vi "TEST - Get Array Element TDEnum.vi"(8 "error in (no error)":errorcluster) -> (0 "error out":errorcluster, 2 "pass":bool)   [LabVIEW 2013]
uses:
  source/library/Type Descriptor Enumeration.ctl
panel:
  out "Failures":T2(array[cluster]) {"result"."Element Type" format="%.0x"; "exected result"."Element Type" format="%.0x"}
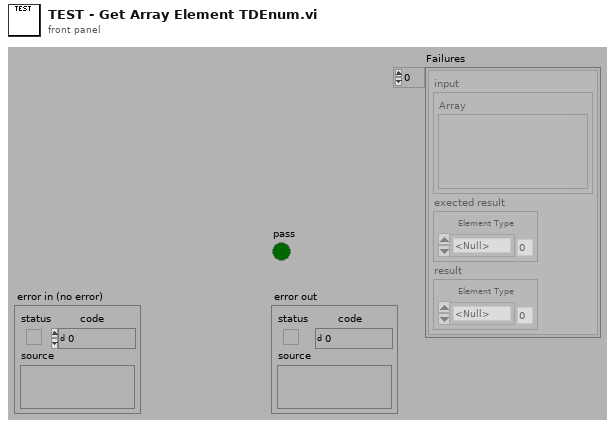
[diagram p1: front panel]
types:
  T1 = typedef "Type Descriptor Enumeration.ctl" = enum8{"<Null>", "I8", "I16", "I32", "I64", "U8", "U16", "U32", "U64", "SGL", "DBL", "EXT", "CSG", "CDB", "CXT", "0x0F", "0x10", "0x11", "0x12", "0x13", "0x14", "Enum U8", "Enum U16", "Enum U32", "Enum U64", "SGL PQ", "DBL PQ", "EXT PQ", "CSG PQ", "CDB PQ", "CXT PQ", "0x1F", "0x20", "Boolean", "0x22", "0x23", "0x24", "0x25", "0x26", "0x27", "0x28", "0x29", "0x2A", "0x2B", "0x2C", "0x2D", "0x2E", "0x2F", "String", "0x31", "Path", "Pict", "0x34", "0x35", "0x36", "DAQ", "0x38", "0x39", "0x3A", "0x3B", "0x3C", "0x3D", "0x3E", "0x3F", "Array", "0x41", "0x42", "0x43", "0x44", "0x45", "0x46", "0x47", "0x48", "0x49", "0x4A", "0x4B", "0x4C", "0x4D", "0x4E", "0x4F", "Cluster", "0x51", "0x52", "Variant", "Waveform", "0x55", "0x56", "0x57", "0x58", "0x59", "0x5A", "0x5B", "0x5C", "0x5D", "0x5E", "0x5F", "0x60", "0x61", "0x62", "0x63", "0x64", "0x65", "0x66", "0x67", "0x68", "0x69", "0x6A", "0x6B", "0x6C", "0x6D", "0x6E", "0x6F", "Refnum"}
  T2 = cluster{"input":cluster{"Array":variant}, "exected result":cluster{"Element Type":T1}, "result":cluster{"Element Type":T1}}[]
  T3 = typedef "Type Descriptor Header.ctl" = cluster{"length":u16, "private":u8, "type":T1, "# elements":u16}
  T4 = cluster{"input":cluster{"Array":variant}, "exected result":cluster{"Element Type":T1}, "result":cluster{"Element Type":T1}}
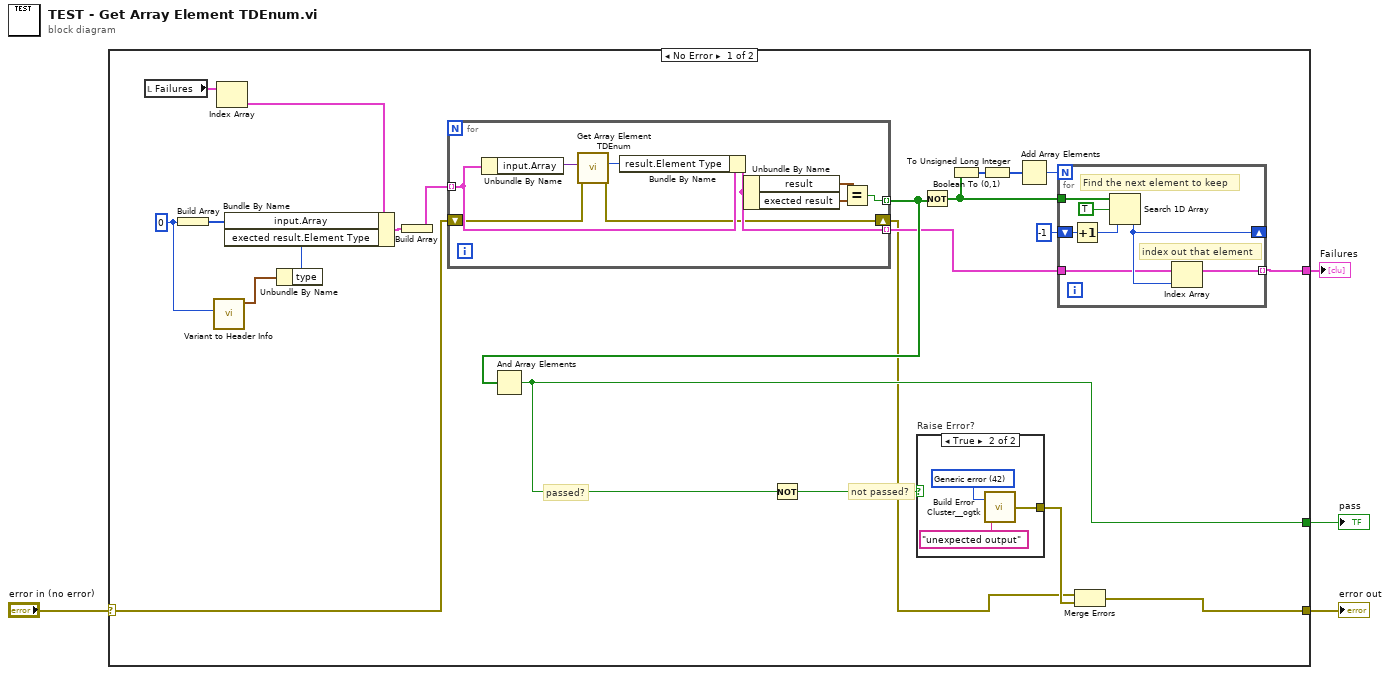
[diagram p0: block diagram]
diagram:
  n1 = case shown="No Error" "error in (no error)" {
    selector: "error in (no error)" -> [w12 w46]
    tunnel: [w23 _] -> w4
    tunnel: [w26 w46] -> w2
    tunnel: [w15 _] -> w1
    frame No Error {
      w6 = 0
      # "not passed?"
      # "passed?"
      n2 = local read "Failures"() -> (w10:T2)
      n3 = Build Array(w6) -> (w8:i32[])
      n4 = call "Variant to Header Info.vi"("Variant"=w6) -> ("Type Descriptor Header"=w7:T3)  [unwired: 3 in, 2 out]
      n5 = Index Array(array=w10) -> (element=w9:T4)  [unwired: 1 in]
      n6 = Unbundle By Name(w7) -> ("type"=w5:T1)
      n7 = Bundle By Name(cluster=w9, "input.Array"=w8, "exected result.Element Type"=w5) -> (w14:T4)
      n8 = Build Array(w14) -> (w13:T2)
      n9 = for {
        tunnel: w13 -> [w41] mode=indexing
        tunnel: [w42] -> w17 mode=indexing
        tunnel: [w40] -> w16 mode=indexing
        shift-right: [w34] -> w11
        shift-left: w12 -> [w35]
        n10 = Unbundle By Name(w41) -> ("input.Array"=w37:variant)
        n11 = call "Get Array Element TDEnum.vi"("error in (no error)"=w35, "Array"=w37) -> ("error out"=w34:errorcluster, "Element Type"=w36:T1)  [unwired: 8 in]
        n12 = Bundle By Name(cluster=w41, "result.Element Type"=w36) -> (w40:T4)
        n13 = Unbundle By Name(w40) -> ("result"=w39:cluster{"Element Type":T1}, "exected result"=w38:cluster{"Element Type":T1})
        n14 = Equal?(x=w39, y=w38) -> (x = y?=w42:bool)
      }
      n15 = And Array Elements(Boolean array=w17) -> (logical AND=w23:bool)
      n16 = Not(x=w23) -> (.not. x?=w24:bool)
      n17 = case "Raise Error?" shown="True" w24 {
        tunnel: [_ w43] -> w25
        frame False {
        }
        frame True {
          w44 = 42 items=["No error", "Argument error", "Memory is full", "Out of zone", "End of file", "File already open", "Generic file I/O error", "File not found", "File permission error", "Disk is full", "Duplicate path", "Too many files open", "System feature not enabled", "Resource file not found", "Cannot add resource", "Resource not found", "Image not found", "Image memory error", "Pen does not exist", "Config type invalid", "Config token not found", "Config parse error", "Config memory error", "Bad external code format", "Bad external code offset", "External code not present", "Null window", "Destroy window error", "Null menu", "Print aborted", "Bad print record", "Print driver error", "Windows error during printing", "Memory error during printing", "Print dialog error", "Generic print error", "Invalid device refnum", "Device not found", "Device parameter error", "Device unit error", "Cannot open device", "Device call aborted", "Generic error", "Cancelled by user", "Object ID too low", "Object ID too high", "Object not in heap", "Unknown heap", "Unknown object (invalid DefProc)", "Unknown object (DefProc not in table)", "Message out of range", "Invalid (null) method", "Unknown message", "Manager call not supported", "Bad address", "Network operation in progress", "Network operation timed out", "Connection is busy", "Network attribute not supported", "Network error", "Address in use", "System out of memory", "Connection aborted", "Connection refused", "Not connected", "Already connected", "Connection closed", "Initialization error (interapplication manager)", "Bad occurrence", "Wait on unbound occurrence handler", "Occurrence queue overflow", "Datalog type conflict", "Unused", "Unrecognized type (interapplication manager)", "Memory corrupt", "Failed to make temporary DLL", "Old CIN version", "Drag socket not found", "Failed to load drop-object", "Failed to register OLE object", "Failed to release OLE object", "Format specifier type mismatch", "Unknown format specifier", "Too few format specifiers", "Too many format specifiers", "Scan failed", "Newer CIN version", "Error converting to variant", "Runtime menu error", "Password tampered", "Variant attribute not found", "Incompatible variant data type", "Event data is not available", "Event Store is not present", "Occurrence is not found", "Event Queue is not created", "Event info is not available", "Refnum passed is NULL", "Error retrieving Class GUID", "Error retrieving CoClass GUID", "Error retrieving TypeLib GUID.", "Bad built application magic bytes.", "Specific driver is different from the specific driver associated with the Logical Name.", "There is no session opened to the class driver.", "Max Error", "MAX - Error with config objects", "MAX - Error loading configuration", "MAX - Group not supported"]
          n18 = call <userlib>:"Build Error Cluster__ogtk.vi"("String to Prepend to source (\"\")"="unexpected output" ("String to Prepend to source (\"\")"), "code"=w44) -> ("error out"=w43:errorcluster)
        }
      }
      n19 = Not(x=w17) -> (.not. x?=w19:bool[])
      n20 = Boolean To (0,1)(Boolean=w19) -> (0, 1=w20:i16[])
      n21 = To Unsigned Long Integer(number=w20) -> (unsigned 32bit integer=w18:u32[])
      n22 = Add Array Elements(numeric array=w18) -> (sum=w21:u32)
      n23 = for {
        N: w21 -> [_]
        tunnel: w16 -> [w29]
        tunnel: w19 -> [w33]
        shift-right: [w30] -> _
        shift-left: -1 ("start index (0)") -> [w31]
        tunnel: [w28] -> w15 mode=indexing
        # "index out that element"
        # "Find the next element to keep"
        n24 = Increment(x=w31) -> (x+1=w27:i32)
        n25 = Search 1D Array(1D array=w33, element=TRUE, start index (0)=w27) -> (index of element=w30:i32)
        n26 = Index Array(array=w29, index=w30) -> (element=w28:T4)
      }
      n27 = Merge Errors(w11, w25) -> (w26:errorcluster)
    }
    frame Error {
    }
  }
  "pass" <- w4
  "error out" <- w2
  "Failures" <- w1
